vi "SetPosTables.vi"(8 "Error in (no err)":errorcluster caption="entrée d'erreur (pas d'erreur)", 9 "ScanFunc":i32, 10 "SinglePar":bool, 11 "Experiment In":refnum<class "Experiment.lvclass"> caption="DNL_LabVIEW Object in") -> (0 "error out":errorcluster caption="sortie d'erreur", 2 "NbPos":i32, 3 "Experiment Out":refnum<class "Experiment.lvclass"> caption="DNL_LabVIEW Object out")   [LabVIEW 2019, in "Experiment.lvclass"]
uses:
  Experiment.lvclass
  Experiment.lvclass/Experiment.ctl
  DevicesClass/BaseDevice/BaseDevice.lvclass
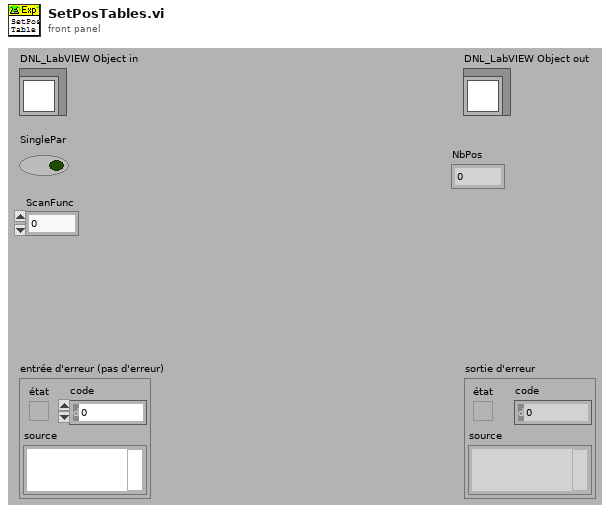
[diagram p1: front panel]
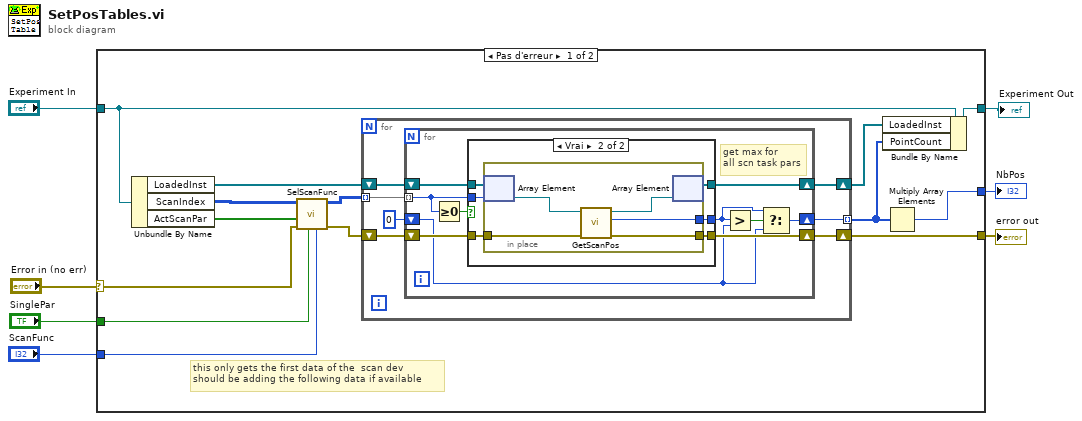
[diagram p0: block diagram]
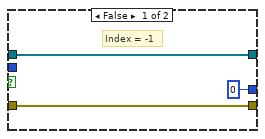
[diagram p2: hidden frame]
diagram:
  n1 = case shown="Pas d'erreur" "Error in (no err)" {
    selector: "Error in (no err)" -> [w12 w54]
    tunnel: [w17 w54] -> w6
    tunnel: [w19 w53] -> w4
    tunnel: "Experiment In" -> [w21 w53]
    tunnel: [w15 _] -> w3
    tunnel: "ScanFunc" -> [w10 _]
    tunnel: "SinglePar" -> [w11 _]
    frame No Error {
      # "this only gets the first data of the  scan dev\nshould be adding the following data if available"
      n2 = Unbundle By Name(w21) -> ("LoadedInst"=w20:refnum<class "BaseDevice.lvclass">[], "ScanIndex"=w14:i32[][], "ActScanPar"=w13:bool[])
      n3 = call "SelScanFunc.vi"("Function"=w10, "SInglePar"=w11, "ErrorIn(No Error)"=w12, "Active ScanPar"=w13, "ScanIndexIn"=w14) -> ("sortie d'erreur"=w9:errorcluster, "ScanIndexOut"=w8:i32[][])  [unwired: 4 in, 1 out]
      n4 = for {
        tunnel: [w23] -> w16 mode=indexing
        tunnel: w8 -> [w26] mode=indexing
        shift-right: [w25] -> w18
        shift-left: w20 -> [w28]
        shift-right: [w24] -> w17
        shift-left: w9 -> [w27]
        n5 = for {
          tunnel: w26 -> [w30] mode=indexing
          shift-right: [w37] -> w25
          shift-left: w28 -> [w38]
          shift-right: [w35] -> w24
          shift-left: w27 -> [w36]
          shift-right: [w32] -> w23
          shift-left: 0 ("nb pos") -> [w29]
          # "get max for \nall scn task pars"
          n6 = Greater Or Equal To 0?(x=w30) -> (x >= 0?=w31:bool)
          n7 = case shown="Vrai" w31 {
            tunnel: w38 -> [w41 w47]
            tunnel: w30 -> [_ w46]
            tunnel: [w41 w45] -> w37
            tunnel: w36 -> [w40 w44]
            tunnel: [w40 w43] -> w35
            tunnel: [0 ("nb pos") w42] -> w33
            frame False {
              # "Index = -1"
            }
            frame True {
              n8 = in-place {
                in-place-border: w44 -> [w51]
                in-place-border: [w48] -> w42
                in-place-border: [w50] -> w43
                n9 = in-place-array #1(w47, w46) -> (w52:refnum<class "BaseDevice.lvclass">)
                n10 = call "GetScanPos.vi"("error in (no error)"=w51, "BaseDevice en entrée"=w52) -> ("error out"=w50:errorcluster, "nb pos"=w48:i32, "BaseDevice en sortie"=w49:refnum<class "BaseDevice.lvclass">)  [unwired: 4 in, 3 out]
                n11 = in-place-array #1(w49) -> (w45:refnum<class "BaseDevice.lvclass">[])  [unwired: 1 out]
              }
            }
          }
          n12 = Greater?(x=w33, y=w29) -> (0:w34:bool)
          n13 = Select(t=w33, s=w34, f=w29) -> (s? t:f=w32:i32)
        }
      }
      n14 = Bundle By Name(cluster=w21, "LoadedInst"=w18, "PointCount"=w16) -> (w19:refnum<class "Experiment.lvclass">)
      n15 = Multiply Array Elements(1:w16) -> (0:w15:i32)
    }
    frame Error {
    }
  }
  "error out" <- w6
  "Experiment Out" <- w4
  "NbPos" <- w3
